vi "ex_TCP Query.vi"(0 "TCP Network Connection in":refnum<k5>, 2 "Termination character":string="\n", 7 "Query string":string, 11 "error in (no error)":errorcluster, 12 "Initial byte timeout ms (1000)":i32=1000) -> (4 "TCP Network Connection out":refnum<k5>, 8 "Message data out":string, 10 "Warning":bool, 15 "error out":errorcluster)   [LabVIEW 2013]
doc: "Query and Read will issue a query string over TCP Write, then attempt to retrieve the responce message with minimal recovery time in case of dropped connections/unexpected message lengths.\n\nShould be tweaked to suit expected communicaton specifics.."
panel:
  out "substring":string
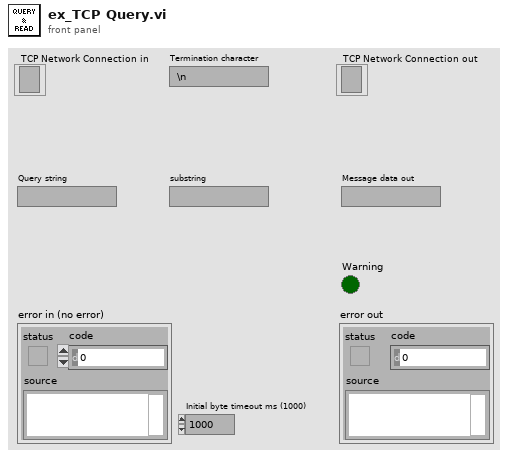
[diagram p1: front panel]
types:
  T1 = enum16{"Standard", "Buffered", "CRLF", "Immediate"}
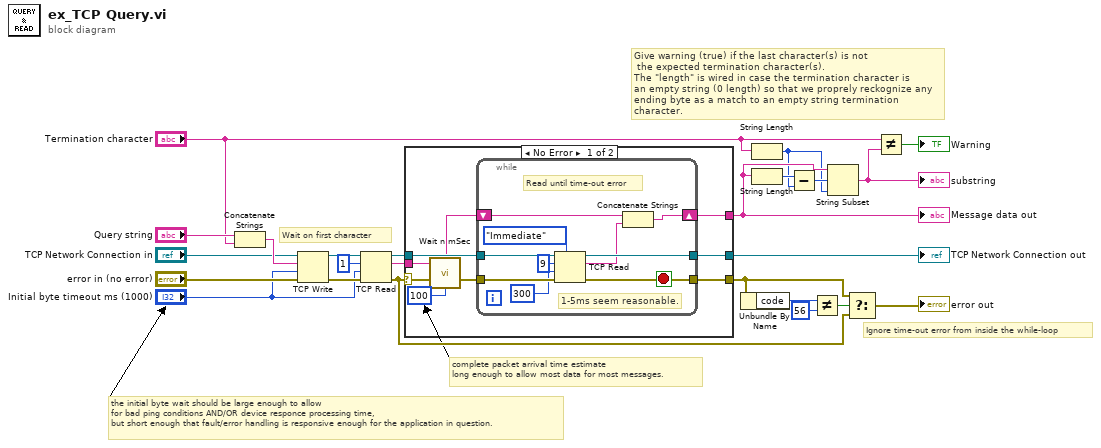
[diagram p0: block diagram]
diagram:
  # "the initial byte wait should be large enough to allow\nfor bad ping conditions AND/OR device responce processing time,\nbut short enough that fault/error handling is responsive enough for the application in question."
  # "complete packet arrival time estimate \nlong enough to allow most data for most messages."
  # "Ignore time-out error from inside the while-loop"
  # "Give warning (true) if the last character(s) is not\n the expected termination character(s).\nThe \"length\" is wired in case the termination character is\nan empty string (0 length) so that we proprely reckognize any\nending byte as a match to an empty string termination character."
  # "Wait on first character"
  n1 = Concatenate Strings("Query string", "Termination character") -> (w24:string)
  n2 = TCP Write(connection ID="TCP Network Connection in", data in=w24, error in (no error)="error in (no error)", 9:"Initial byte timeout ms (1000)") -> (connection ID out=w17:refnum<k5>, error out=w18:errorcluster)  [unwired: 1 out]
  n3 = TCP Read(connection ID=w17, bytes to read=1, error in (no error)=w18, 9:"Initial byte timeout ms (1000)") -> (connection ID out=w16:refnum<k5>, data out=w15:string, error out=w5:errorcluster)  [unwired: 1 in]
  n4 = case shown="No Error" w5 {
    selector: w5 -> [w25 w43]
    tunnel: [w32 w45] -> w22
    tunnel: [w31 w43] -> w6
    tunnel: w16 -> [w30 w45]
    tunnel: w15 -> [w27 w44]
    tunnel: [w26 w44] -> w14
    frame No Error {
      n5 = call "Wait n mSec.vi"("Error in (no error)"=w25, "Milliseconds to Wait (1)"=u32 100) -> ("Error Out"=w29:errorcluster)  [unwired: 13 in]
      n6 = while {
        tunnel: [w42] -> w32
        tunnel: [w34] -> w31
        tunnel: w30 -> [w40]
        tunnel: w29 -> [w39]
        shift-right: [w35] -> w26
        shift-left: w27 -> [w37]
        stop <- w34 stop-if-true
        # "1-5ms seem reasonable."
        # "Read until time-out error"
        n7 = TCP Read(connection ID=w40, bytes to read=9, error in (no error)=w39, 7:T1."Immediate" ("mode (standard)"), 9:300 ("timeout ms (25000)")) -> (connection ID out=w42:refnum<k5>, data out=w36:string, error out=w34:errorcluster)
        n8 = Concatenate Strings(w37, w36) -> (w35:string)
      }
    }
    frame Error {
    }
  }
  "Message data out" <- w14
  "TCP Network Connection out" <- w22
  n9 = Unbundle By Name(w6) -> ("code"=w10:i32)
  n10 = String Length(string="Termination character") -> (length=w1:i32)
  n11 = String Length(string=w14) -> (length=w4:i32)
  n12 = Subtract(x=w4, y=w1) -> (x-y=w2:i32)
  n13 = Not Equal?(x=w10, y=56) -> (x != y?=w8:bool)
  n14 = String Subset(string=w14, offset (0)=w2, length (rest)=w1) -> (substring=w12:string)
  "substring" <- w12
  n15 = Select(t=w6, s=w8, f=w5) -> (s? t:f=→"error out":errorcluster)
  n16 = Not Equal?(x="Termination character", y=w12) -> (x != y?=→"Warning":bool)
